vi "testvi.vi"   [LabVIEW 2017]
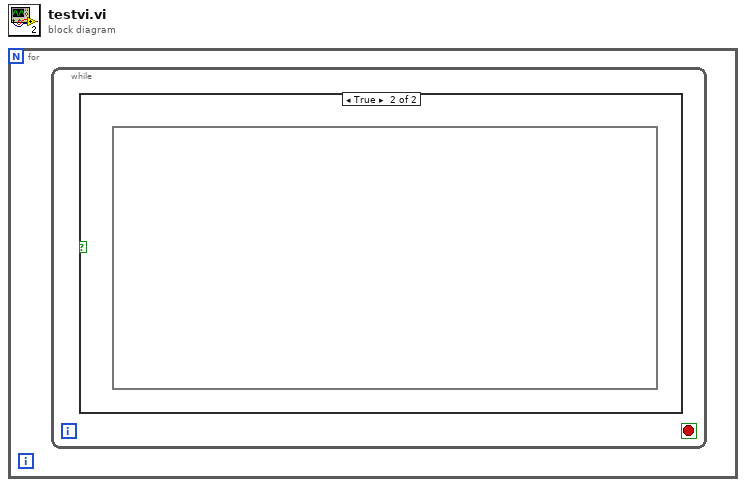
[diagram p0: block diagram]
diagram:
  n1 = for {
    n2 = while {
      stop <- _ stop-if-true
      n3 = case shown="True" {
        selector: _ -> [_ _]
        frame False {
        }
        frame True {
          n4 = formula code=""() -> ()
        }
      }
    }
  }
